vi "Read Logger.vi"(8 "error in (no error)":errorcluster, 11 "LoggingActor in":refnum<class "LoggingActor.lvclass">) -> (0 "error out":errorcluster, 2 "Logger":refnum<class "Logger.lvclass">, 3 "LoggingActor out":refnum<class "LoggingActor.lvclass">)   [LabVIEW 2022 SP3, in "LoggingActor.lvlib" / "LoggingActor.lvclass"]
uses:
  LoggingActor.lvclass
  LoggingActor.lvclass/LoggingActor.ctl
  Logger/Source/Logger/Logger.lvclass
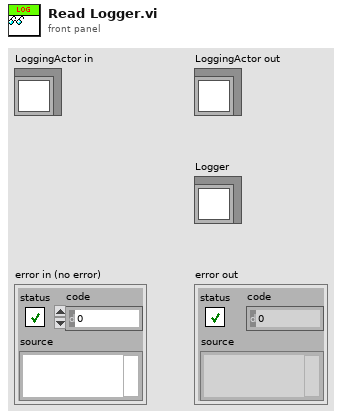
[diagram p1: front panel]
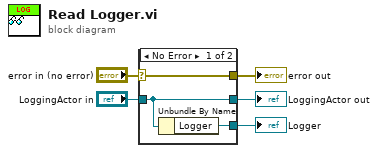
[diagram p0: block diagram]
diagram:
  n1 = case shown="No Error" "error in (no error)" {
    selector: "error in (no error)" -> [w8 w9]
    tunnel: [w8 w9] -> w4
    tunnel: [w7 w10] -> w2
    tunnel: "LoggingActor in" -> [w7 w10]
    tunnel: [w6 _] -> w1
    frame No Error {
      n2 = Unbundle By Name(w7) -> ("Logger"=w6:refnum<class "Logger.lvclass">)
    }
    frame Error {
    }
  }
  "error out" <- w4
  "LoggingActor out" <- w2
  "Logger" <- w1
